vi "Example Callback.vi"() -> ()   [LabVIEW 2010]
uses:
  C:/tf/play/labview/Tinkerforge.dll
  Tinkerforge.dll
panel:
  in  "stop":bool
  out "voltage (V)":sgl format="%#_13g"
  in  "uid":string="amb"
  in  "port":i32=4223
  in  "host":string="localhost"
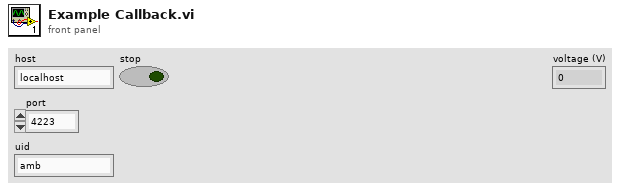
[diagram p1: front panel]
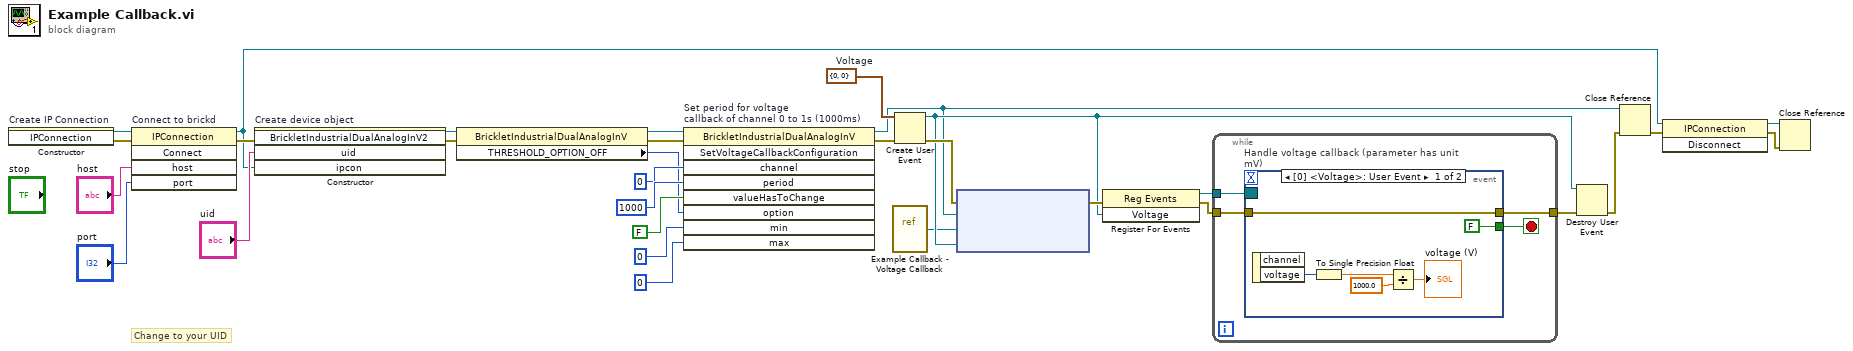
[diagram p0: block diagram]
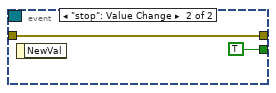
[diagram p2: hidden frame]
diagram:
  w15 = cluster{"channel":u8, "voltage":i32} {"channel"=0, "voltage"=0}  # Voltage
  # "Change to your UID"
  n1 = constructor on="Create IP Connection" class="IPConnection"() -> (reference out=w31:refnum<k24>, error out=w12:errorcluster)  [unwired: 3 in, 1 out]
  n2 = invoke on="Connect to brickd" class="IPConnection" method="Connect"(reference=w31, error in=w12, "host"="host", "port"="port") -> (reference out=w24:refnum<k24>, error out=w27:errorcluster)  [unwired: 1 in, 3 out]
  n3 = constructor on="Create device object" class="BrickletIndustrialDualAnalogInV"(error in=w27, "uid"="uid", "ipcon"=w24) -> (reference out=w6:refnum<k24>, error out=w3:errorcluster)  [unwired: 2 in, 3 out]
  n4 = property class="BrickletIndustrialDualAnalogInV"(reference=w6, error in=w3) -> (reference out=w5:refnum<k24>, error out=w4:errorcluster, "THRESHOLD_OPTION_OFF"=w1:u16)
  n5 = invoke on="Set period for voltage\ncallback of channel 0 to 1s (1000ms)" class="BrickletIndustrialDualAnalogInV" method="SetVoltageCallbackConfiguration"(reference=w5, error in=w4, "channel"=u8 0 ("sensor"), "period"=i64 1000, "valueHasToChange"=FALSE, "option"=w1, "min"=0, "max"=0) -> (reference out=w13:refnum<k24>, error out=w14:errorcluster)  [unwired: 1 in, 7 out]
  n6 = vi-ref "Example Callback - Voltage Callback.vi"() -> ("vi reference"=w2:refnum<vi>)
  n7 = Create User Event(user event datatype=w15, error in=w14) -> (user event=w17:refnum<user-event>, error out=w22:errorcluster)
  n8 = node ("Register Event Callback")(w22, w13, w2, w17) -> (w21:errorcluster)  [unwired: 1 in, 1 out]
  n9 = register-events(error in=w21, w17) -> (reference out=w20:refnum<event-registration>, error out=w18:errorcluster)  [unwired: 1 in]
  n10 = while {
    tunnel: w20 -> [w35]
    tunnel: [w34] -> w19
    tunnel: w18 -> [w33]
    stop <- w32 stop-if-true
    n11 = event "Handle voltage callback (parameter has unit mV)" shown="[0] <Voltage>: User Event" {
      selector: w35 -> [_ _]
      dyn-events: _ -> [_ _]
      timeout: _ -> [_ _]
      tunnel: [w38 w42] -> w34
      tunnel: w33 -> [w38 w42]
      tunnel: [FALSE TRUE] -> w32
      event User Event {
        n12 = event-data() -> ("voltage"=w39:i32)  [unwired: 1 in, 1 out]
        n13 = To Single Precision Float(number=w39) -> (single precision float=w40:sgl)
        n14 = Divide(x=w40, y=sgl 1000.0) -> (x/y=→"voltage (V)":sgl)
      }
      event "stop": Value Change {
        n15 = event-data() -> ()  [unwired: 1 in, 1 out]
      }
    }
  }
  n16 = Destroy User Event(user event=w17, error in=w19) -> (error out=w16:errorcluster)
  n17 = Close Reference(reference=w13, error in (no error)=w16) -> (error out=w26:errorcluster)
  n18 = invoke class="IPConnection" method="Disconnect"(reference=w24, error in=w26) -> (reference out=w23:refnum<k24>, error out=w25:errorcluster)  [unwired: 1 in, 1 out]
  n19 = Close Reference(reference=w23, error in (no error)=w25) -> ()  [unwired: 1 out]
